vi "Remove Bitfile.vi"(8 "error in (no error)":errorcluster, 10 "RIO name":string, 11 "Item Ref in":T1 format="%.0x") -> (0 "error out":errorcluster, 3 "Item Ref out":T1 format="%.0x")   [LabVIEW 2015, in "Engine Simulation Toolkit System Explorer.lvlib"]
uses:
  Engine Simulation Toolkit System Explorer.lvlib
  <vilib>/NI Veristand/Custom Device API/Custom Device Item Ref.ctl
  Shared/Constants and GUIDs.vi
  <vilib>/NI Veristand/Custom Device Tools/Custom Device Utility Library/NI VeriStand - Search for Item by GUID.vi
  <vilib>/NI Veristand/Custom Device API/Custom Device API.lvlib
  <vilib>/NI Veristand/Custom Device Tools/Custom Device Utility Library/Custom Device Utility Library.lvlib
  Shared/Engine Simulation Toolkit Shared.lvlib
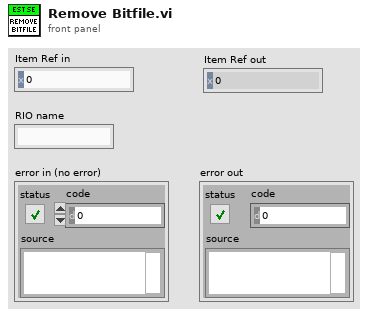
[diagram p1: front panel]
types:
  T1 = typedef "Custom Device API.lvlib/Custom Device Item Ref.ctl" = u64
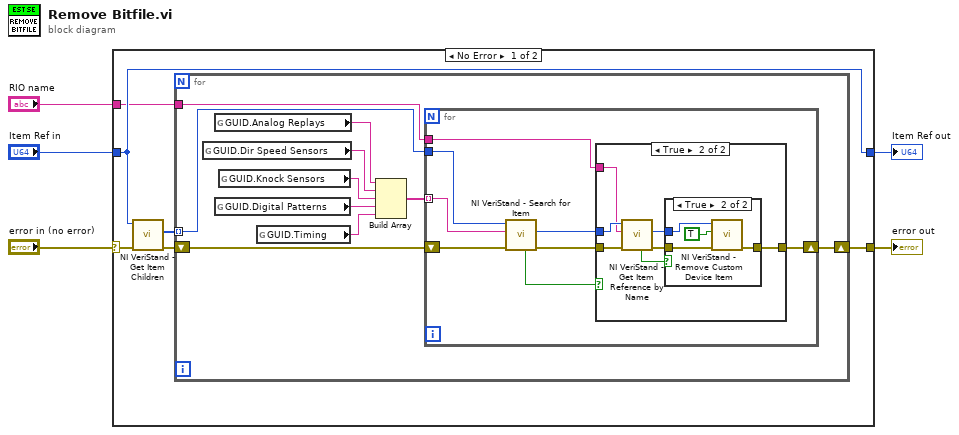
[diagram p0: block diagram]
diagram:
  n1 = case shown="No Error" "error in (no error)" {
    selector: "error in (no error)" -> [w11 w44]
    tunnel: [w8 w44] -> w3
    tunnel: "Item Ref in" -> [w7 w43]
    tunnel: "RIO name" -> [w6 _]
    tunnel: [w7 w43] -> w1
    frame No Error {
      n2 = call <vilib>:"NI VeriStand - Get Item Children.vi"("error in (no error)"=w11, "Item Ref in"=w7) -> ("error out"=w9:errorcluster, "Child Refs"=w10:T1[])  [unwired: 6 in, 2 out]
      n3 = for {
        tunnel: w10 -> [w21] mode=indexing
        shift-right: [w14] -> w8
        shift-left: w9 -> [w20]
        tunnel: w6 -> [w13]
        n4 = global read "Constants and GUIDs.vi" "GUID.Dir Speed Sensors"() -> (w18:string)
        n5 = global read "Constants and GUIDs.vi" "GUID.Analog Replays"() -> (w19:string)
        n6 = global read "Constants and GUIDs.vi" "GUID.Digital Patterns"() -> (w16:string)
        n7 = global read "Constants and GUIDs.vi" "GUID.Knock Sensors"() -> (w17:string)
        n8 = global read "Constants and GUIDs.vi" "GUID.Timing"() -> (w12:string)
        n9 = Build Array(w19, w18, w17, w16, w12) -> (w15:string[])
        n10 = for {
          tunnel: w21 -> [w29]
          tunnel: w15 -> [w25] mode=indexing
          shift-right: [w24] -> w14
          shift-left: w20 -> [w28]
          tunnel: w13 -> [w23]
          n11 = call-poly <vilib>:"NI VeriStand - Search for Item.vi"("error in"=w28, "Item GUID"=w25, "Section Ref in"=w29) -> ("error out"=w27:errorcluster, "Item Ref"=w26:T1, "Found"=w22:bool)  [unwired: 5 in, 1 out]
          n12 = case shown="True" w22 {
            tunnel: w27 -> [w30 w37]
            tunnel: w26 -> [_ w36]
            tunnel: [w30 w33] -> w24
            tunnel: w23 -> [_ w32]
            frame False {
            }
            frame True {
              n13 = call <vilib>:"NI VeriStand - Get Item Reference by Name.vi"("error in (no error)"=w37, "Item Name"=w32, "Parent Ref in"=w36) -> ("error out"=w35:errorcluster, "Item Ref"=w34:T1, "Found"=w31:bool)  [unwired: 5 in, 1 out]
              n14 = case shown="True" w31 {
                tunnel: w35 -> [w38 w42]
                tunnel: w34 -> [_ w41]
                tunnel: [w38 w40] -> w33
                frame False {
                }
                frame True {
                  n15 = call <vilib>:"NI VeriStand - Remove Custom Device Item.vi"("error in (no error)"=w42, "Force Delete (F)"=TRUE, "Item Ref in"=w41) -> ("error out"=w40:errorcluster)  [unwired: 7 in, 1 out]
                }
              }
            }
          }
        }
      }
    }
    frame Error {
    }
  }
  "error out" <- w3
  "Item Ref out" <- w1
